vi "exponential fit.vi"() -> ()   [LabVIEW 2015]
uses:
  <vilib>/Utility/file.llb/Read Delimited Spreadsheet (DBL).vi
  <vilib>/Analysis/NI_AALPro.lvlib
  <vilib>/Analysis/NI_AALBase.lvlib
panel:
  out "Half Life (s)":dbl=-79.0458411255295
  out "Decay Plot":T1(graph)=[{"Best Exponential Fit"=[0.0, 1.0, 2.0, 3.0, 4.0, 5.0, 6.0, 7.0, 8.0, 9.0, 10.0, 11.0, 12.0, 13.0, 14.0, 15.0, 16.0, 17.0, 18.0, 19.0, 20.0, 21.0, 22.0, 23.0, 24.0, 25.0, 26.0, 27.0, 28.0, 29.0, 30.0, 31.0, 32.0, 33.0, 34.0, 35.0, 36.0, 37.0, 38.0, 39.0, 40.0, 41.0, 42.0, 43.0, 44.0, 45.0, 46.0, 47.0, 48.0, 49.0, 50.0, 51.0, 52.0, 53.0, 54.0, 55.0, 56.0, 57.0, 58.0, 59.0, 60.0, 61.0, 62.0, 63.0, 64.0, 65.0, 66.0, 67.0, 68.0, 69.0, 70.0, 71.0, 72.0, 73.0, 74.0, 75.0, 76.0, 77.0, 78.0, 79.0, 80.0, 81.0, 82.0, 83.0, 84.0, 85.0, 86.0, 87.0, 88.0, 89.0, 90.0, 91.0, 92.0, 93.0, 94.0, 95.0, 96.0, 97.0, 98.0, 99.0, 100.0, 101.0, 102.0, 103.0, 104.0, 105.0, 106.0, 107.0, 108.0, 109.0, 110.0, 111.0, 112.0, 113.0, 114.0, 115.0, 116.0, 117.0, 118.0, 119.0, 120.0, 121.0, 122.0, 123.0, 124.0, 125.0, 126.0, 127.0, 128.0, 129.0, 130.0, 131.0, 132.0, 133.0, 134.0, 135.0, 136.0, 137.0, 138.0, 139.0, 140.0, 141.0, 142.0, 143.0, 144.0, 145.0, 146.0, 147.0, 148.0, 149.0, 150.0, 151.0, 152.0, 153.0, 154.0, 155.0, 156.0, 157.0, 158.0, 159.0, 160.0, 161.0, 162.0, 163.0, 164.0, 165.0, 166.0, 167.0, 168.0, 169.0, 170.0, 171.0, 172.0, 173.0, 174.0, 175.0, 176.0, 177.0, 178.0, 179.0, 180.0, 181.0, 182.0, 183.0, 184.0, 185.0, 186.0, 187.0, 188.0, 189.0, 190.0, 191.0, 192.0, 193.0, 194.0, 195.0, 196.0, 197.0, 198.0, 199.0, 200.0, 201.0, 202.0, 203.0, 204.0, 205.0, 206.0, 207.0, 208.0, 209.0, 210.0, 211.0, 212.0, 213.0, 214.0, 215.0, 216.0, 217.0, 218.0, 219.0, 220.0, 221.0, 222.0, 223.0, 224.0, 225.0, 226.0, 227.0, 228.0, 229.0, 230.0, 231.0, 232.0, 233.0, 234.0, 235.0, 236.0, 237.0, 238.0, 239.0, 240.0, 241.0, 242.0, 243.0, 244.0, 245.0, 246.0, 247.0, 248.0, 249.0, 250.0, 251.0, 252.0, 253.0, 254.0, 255.0, 256.0, 257.0, 258.0, 259.0, 260.0, 261.0, 262.0, 263.0, 264.0, 265.0, 266.0, 267.0, 268.0, 269.0, 270.0, 271.0, 272.0, 273.0, 274.0, 275.0, 276.0, 277.0, 278.0, 279.0, 280.0, 281.0, 282.0, 283.0, 284.0, 285.0, 286.0, 287.0, 288.0, 289.0, 290.0, 291.0, 292.0, 293.0, 294.0, 295.0, 296.0, 297.0, 298.0, 299.0, 300.0], "all rows"=[0.0, 37.0, 51.0, 62.0, 64.0, 69.0, 55.0, 70.0, 52.0, 84.0, 66.0, 49.0, 62.0, 61.0, 55.0, 68.0, 51.0, 56.0, 55.0, 60.0, 46.0, 62.0, 45.0, 56.0, 63.0, 59.0, 49.0, 58.0, 53.0, 57.0, 63.0, 48.0, 55.0, 55.0, 49.0, 65.0, 45.0, 51.0, 39.0, 46.0, 45.0, 49.0, 47.0, 36.0, 56.0, 43.0, 55.0, 38.0, 37.0, 48.0, 48.0, 43.0, 57.0, 45.0, 37.0, 36.0, 47.0, 37.0, 28.0, 30.0, 42.0, 41.0, 39.0, 36.0, 42.0, 38.0, 39.0, 39.0, 32.0, 31.0, 33.0, 29.0, 37.0, 37.0, 27.0, 29.0, 24.0, 32.0, 31.0, 30.0, 37.0, 22.0, 41.0, 32.0, 32.0, 31.0, 33.0, 33.0, 30.0, 30.0, 30.0, 27.0, 19.0, 33.0, 27.0, 30.0, 27.0, 28.0, 29.0, 36.0, 35.0, 33.0, 22.0, 31.0, 12.0, 19.0, 14.0, 29.0, 28.0, 15.0, 17.0, 25.0, 18.0, 22.0, 26.0, 25.0, 17.0, 21.0, 20.0, 27.0, 21.0, 20.0, 20.0, 23.0, 31.0, 25.0, 24.0, 22.0, 14.0, 17.0, 13.0, 25.0, 16.0, 20.0, 28.0, 14.0, 23.0, 21.0, 23.0, 18.0, 26.0, 18.0, 22.0, 24.0, 10.0, 17.0, 13.0, 15.0, 12.0, 17.0, 19.0, 18.0, 13.0, 14.0, 22.0, 21.0, 12.0, 18.0, 18.0, 13.0, 9.0, 19.0, 21.0, 19.0, 12.0, 16.0, 11.0, 11.0, 14.0, 11.0, 20.0, 12.0, 7.0, 13.0, 9.0, 13.0, 15.0, 14.0, 19.0, 9.0, 13.0, 18.0, 12.0, 9.0, 10.0, 7.0, 9.0, 11.0, 9.0, 8.0, 7.0, 9.0, 13.0, 7.0, 23.0, 12.0, 15.0, 11.0, 10.0, 15.0, 6.0, 13.0, 10.0, 8.0, 4.0, 13.0, 15.0, 8.0, 12.0, 8.0, 12.0, 4.0, 10.0, 16.0, 13.0, 12.0, 12.0, 8.0, 6.0, 14.0, 10.0, 7.0, 13.0, 9.0, 10.0, 13.0, 7.0, 12.0, 8.0, 6.0, 3.0, 9.0, 6.0, 8.0, 12.0, 10.0, 7.0, 9.0, 8.0, 11.0, 9.0, 4.0, 1.0, 3.0, 11.0, 4.0, 5.0, 3.0, 8.0, 8.0, 13.0, 4.0, 8.0, 5.0, 6.0, 5.0, 5.0, 4.0, 6.0, 9.0, 6.0, 5.0, 5.0, 4.0, 5.0, 6.0, 3.0, 8.0, 9.0, 6.0, 8.0, 7.0, 4.0, 4.0, 7.0, 9.0, 4.0, 7.0, 4.0, 5.0, 3.0, 8.0, 6.0, 7.0, 5.0, 3.0, 5.0, 6.0, 4.0, 6.0, 6.0, 3.0, 1.0, 5.0, 8.0, 7.0, 3.0, 2.0, 3.0, 6.0, 5.0]}, {"Best Exponential Fit"=[0.0, 1.0, 2.0, 3.0, 4.0, 5.0, 6.0, 7.0, 8.0, 9.0, 10.0, 11.0, 12.0, 13.0, 14.0, 15.0, 16.0, 17.0, 18.0, 19.0, 20.0, 21.0, 22.0, 23.0, 24.0, 25.0, 26.0, 27.0, 28.0, 29.0, 30.0, 31.0, 32.0, 33.0, 34.0, 35.0, 36.0, 37.0, 38.0, 39.0, 40.0, 41.0, 42.0, 43.0, 44.0, 45.0, 46.0, 47.0, 48.0, 49.0, 50.0, 51.0, 52.0, 53.0, 54.0, 55.0, 56.0, 57.0, 58.0, 59.0, 60.0, 61.0, 62.0, 63.0, 64.0, 65.0, 66.0, 67.0, 68.0, 69.0, 70.0, 71.0, 72.0, 73.0, 74.0, 75.0, 76.0, 77.0, 78.0, 79.0, 80.0, 81.0, 82.0, 83.0, 84.0, 85.0, 86.0, 87.0, 88.0, 89.0, 90.0, 91.0, 92.0, 93.0, 94.0, 95.0, 96.0, 97.0, 98.0, 99.0, 100.0, 101.0, 102.0, 103.0, 104.0, 105.0, 106.0, 107.0, 108.0, 109.0, 110.0, 111.0, 112.0, 113.0, 114.0, 115.0, 116.0, 117.0, 118.0, 119.0, 120.0, 121.0, 122.0, 123.0, 124.0, 125.0, 126.0, 127.0, 128.0, 129.0, 130.0, 131.0, 132.0, 133.0, 134.0, 135.0, 136.0, 137.0, 138.0, 139.0, 140.0, 141.0, 142.0, 143.0, 144.0, 145.0, 146.0, 147.0, 148.0, 149.0, 150.0, 151.0, 152.0, 153.0, 154.0, 155.0, 156.0, 157.0, 158.0, 159.0, 160.0, 161.0, 162.0, 163.0, 164.0, 165.0, 166.0, 167.0, 168.0, 169.0, 170.0, 171.0, 172.0, 173.0, 174.0, 175.0, 176.0, 177.0, 178.0, 179.0, 180.0, 181.0, 182.0, 183.0, 184.0, 185.0, 186.0, 187.0, 188.0, 189.0, 190.0, 191.0, 192.0, 193.0, 194.0, 195.0, 196.0, 197.0, 198.0, 199.0, 200.0, 201.0, 202.0, 203.0, 204.0, 205.0, 206.0, 207.0, 208.0, 209.0, 210.0, 211.0, 212.0, 213.0, 214.0, 215.0, 216.0, 217.0, 218.0, 219.0, 220.0, 221.0, 222.0, 223.0, 224.0, 225.0, 226.0, 227.0, 228.0, 229.0, 230.0, 231.0, 232.0, 233.0, 234.0, 235.0, 236.0, 237.0, 238.0, 239.0, 240.0, 241.0, 242.0, 243.0, 244.0, 245.0, 246.0, 247.0, 248.0, 249.0, 250.0, 251.0, 252.0, 253.0, 254.0, 255.0, 256.0, 257.0, 258.0, 259.0, 260.0, 261.0, 262.0, 263.0, 264.0, 265.0, 266.0, 267.0, 268.0, 269.0, 270.0, 271.0, 272.0, 273.0, 274.0, 275.0, 276.0, 277.0, 278.0, 279.0, 280.0, 281.0, 282.0, 283.0, 284.0, 285.0, 286.0, 287.0, 288.0, 289.0, 290.0, 291.0, 292.0, 293.0, 294.0, 295.0, 296.0, 297.0, 298.0, 299.0, 300.0], "all rows"=[64.13781261084702, 63.5778515552424, 63.02277929099237, 62.4725531360556, 61.92713078103027, 61.386470285900664, 60.85053007681219, 60.31926894287464, 59.79264603299326, 59.27062085272752, 58.75315326117729, 58.2402034678963, 57.73173202983239, 57.22769984829459, 56.72806816594664, 56.23279856382675, 55.7418529583934, 55.255193598596954, 54.772783062976735, 54.29458425678358, 53.82056040912744, 53.35067507014988, 52.88489210822131, 52.42317570716263, 51.9654903634912, 51.51180088369078, 51.062072381505345, 50.616270275256525, 50.17436028518449, 49.73630843081198, 49.30208102833139, 48.87164468801474, 48.444966311646056, 48.02201308997645, 47.602752500201134, 47.18715230345869, 46.77518054235202, 46.36680553849099, 45.961995890056606, 45.5607204693863, 45.16294842058041, 44.768649157129566, 44.37779235956271, 43.990347973115696, 43.606286205420254, 43.22557752421314, 42.84819265506523, 42.47410257913049, 42.103278530914565, 41.735691996062904, 41.371314709168146, 41.01011865159666, 40.65207604933406, 40.29715937084954, 39.945341324978855, 39.59659485882577, 39.25089315568183, 38.90820963296433, 38.56851794017224, 38.231791956859986, 37.89800579062894, 37.56713377513646, 37.23915046812222, 36.9140306494519, 36.59174931917791, 36.27228169561693, 35.955603213444455, 35.641689521805766, 35.33051648244354, 35.022060167841694, 34.716296859385544, 34.41320304553794, 34.11275542003135, 33.814930880075764, 33.5197065245822, 33.22705965240172, 32.93696776057986, 32.64940854262626, 32.36435988679942, 32.081799874406435, 31.80170677811755, 31.52405906029545, 31.248835371339144, 30.976014548042297, 30.705575611965884, 30.437497767825064, 30.171760401890133, 29.908343080401455, 29.6472255479982, 29.38838772616083, 29.131809711667145, 28.87747177506188, 28.62535435913957, 28.375438077440727, 28.127703712761132, 27.88213221567412, 27.638704703065812, 27.397402456683064, 27.158206921694173, 26.921099705262083, 26.686062575130116, 26.453077458219944, 26.22212643924194, 25.99319175931753, 25.76625581461369, 25.54130115498924, 25.318310482653082, 25.09726665083406, 24.878152662462483, 24.660951668863124, 24.445646968459673, 24.232222005490456, 24.020660368735403, 23.81094579025409, 23.603062144134853, 23.396993445254783, 23.192723848050534, 22.990237645299924, 22.789519266914095, 22.5905532787403, 22.393324381375056, 22.19781740898775, 22.004017328154415, 21.81190923670179, 21.621478362561408, 21.43271006263369, 21.245589821661973, 21.060103251116406, 20.876236088087477, 20.693974194189344, 20.513303554472618, 20.33421027634673, 20.156680588511637, 19.980700839898894, 19.80625749862196, 19.633337150935677, 19.461926500204818, 19.292012365881643, 19.1235816824924, 18.95662149863264, 18.791118975971358, 18.627061388263773, 18.46443612037273, 18.303230667298713, 18.14343263321824, 17.98502973053069, 17.82800977891349, 17.67236070438547, 17.51807053837847, 17.365127416817018, 17.21351957920602, 17.06323536772649, 16.914263226339084, 16.766591699895518, 16.620209433257738, 16.475105170424754, 16.331267753667138, 16.18868612266904, 16.047349313677696, 15.907246458660419, 15.768366784468851, 15.63069961201061, 15.494234355428098, 15.358960521284528, 15.22486770775703, 15.091945603836784, 14.960183988536187, 14.829572730102917, 14.70010178524083, 14.571761198337706, 14.444541100699707, 14.318431709792536, 14.19342332848921, 14.069506344324399, 13.946671228755278, 13.824908536428856, 13.704208904455646, 13.584563051689733, 13.465961778015094, 13.348395963638168, 13.231856568386588, 13.116334631014038, 13.001821268511183, 12.888307675422622, 12.775785123169783, 12.664244959379758, 12.553678607219965, 12.444077564738649, 12.33543340421113, 12.227737771491745, 12.120982385371464, 12.015159036941126, 11.910259588960184, 11.80627597523103, 11.703200199978731, 11.601024337236193, 11.499740530234723, 11.399340990799846, 11.29981799875247, 11.201163901315239, 11.103371112524059, 11.0064321126448, 10.910339447595062, 10.815085728370983, 10.720663630479093, 10.627065893373075, 10.534285319895478, 10.442314775724295, 10.351147188824374, 10.260775548903611, 10.171192906873902, 10.08239237431679, 9.994367122953799, 9.907110384121347, 9.820615448250305, 9.734875664350048, 9.64988443949703, 9.565635238327836, 9.482121582536637, 9.399337050377044, 9.31727527616832, 9.235929949805886, 9.155294816276106, 9.075363675175318, 8.996130380233053, 8.917588838839418, 8.83973301157661, 8.762556911754515, 8.686054604950373, 8.610220208552438, 8.535047891307654, 8.460531872873242, 8.386666423372251, 8.313445862952936, 8.24086456135202, 8.168916937461757, 8.097597458900772, 8.026900641588663, 7.956821049324283, 7.887353293367743, 7.818492032026039, 7.750231970242311, 7.682567859188677, 7.615494495862627, 7.549006722686946, 7.483099427113111, 7.417767541228186, 7.353006041365104, 7.288809947716384, 7.225174323951217, 7.1620942768358775, 7.099564955857467, 7.0375815528509325, 6.976139301629357, 6.915233477617446, 6.8548593974882435, 6.795012418803012, 6.735687939654249, 6.676881398311831, 6.618588272872233, 6.560804080910827, 6.5035243791372, 6.446744763053503, 6.39046086661575, 6.334668361898104, 6.2793629587600845, 6.224540404516675, 6.1701964836113135, 6.116327017291741, 6.062927863288686, 6.00999491549733, 5.957524103661581, 5.9055113930610945, 5.8539527842010175, 5.802844312504456, 5.7521820480076205, 5.701962095057627, 5.652180592012944, 5.6028337109464665, 5.553917657351147, 5.505428669848236, 5.457363019898041, 5.409717011513234, 5.3624869809746345, 5.315669296549506, 5.2692603582122866, 5.223256597367765, 5.177654476576681, 5.132450489283706, 5.087641159547824, 5.043223041775032, 4.999192720453404, 4.955546809890459, 4.912281953952806, 4.869394825808094, 4.8268821276691805, 4.784740590540557, 4.742966973966982, 4.701558065784304, 4.6605106818724655, 4.619821665910661]}]
  in  "Path 2":path=path "C:/Users/senkoa/Desktop/PHYS434/week8/constant data"
  in  "Path":path=path "C:/Users/senkoa/Desktop/PHYS434/week8/data"
  out "Constant Rate":T2(graph)={"X Values"=[2.0714285714285716, 6.214285714285714, 10.357142857142858, 14.5, 18.642857142857142, 22.785714285714285, 26.928571428571427, 31.071428571428573, 35.214285714285715, 39.357142857142854, 43.5, 47.642857142857146, 51.785714285714285, 55.92857142857143], "Histogram: h(x)"=[1, 0, 0, 0, 0, 1, 2, 21, 13, 30, 27, 14, 10, 2]}
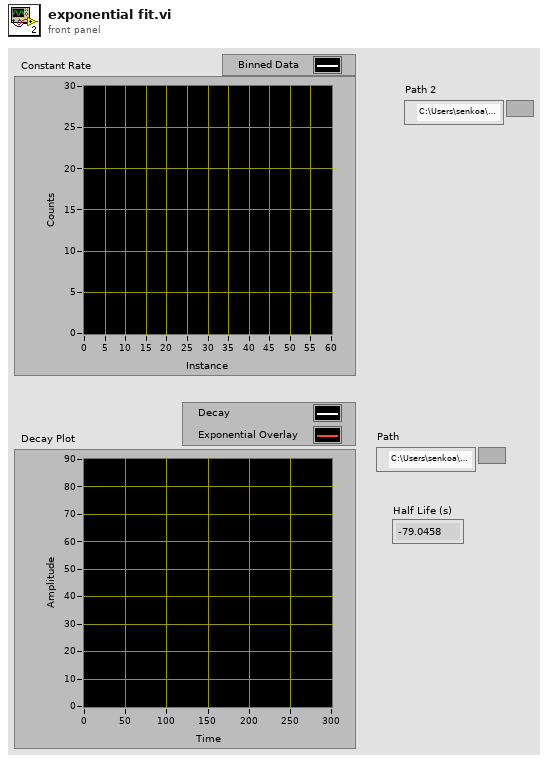
[diagram p1: front panel]
types:
  T1 = cluster{"Best Exponential Fit":dbl[], "all rows":dbl[]}[]
  T2 = cluster{"X Values":dbl[], "Histogram: h(x)":i32[]}
  T3 = cluster{"all rows":dbl[], "Best Exponential Fit":dbl[]}
  T4 = cluster{"all rows":dbl[], "Best Exponential Fit":dbl[]}[]
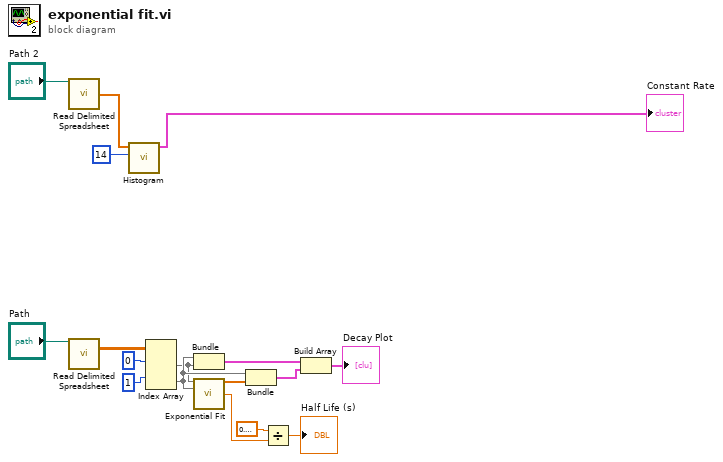
[diagram p0: block diagram]
diagram:
  n1 = call-poly <vilib>:"Read Delimited Spreadsheet.vi"("file path (dialog if empty)"="Path 2") -> ("first row"=w2:dbl[])  [unwired: 9 in, 5 out]
  n2 = call-poly <vilib>:"Read Delimited Spreadsheet.vi"("file path (dialog if empty)"="Path") -> ("all rows"=w15:dbl[][])  [unwired: 9 in, 5 out]
  n3 = call <vilib>:"Histogram.vi"("intervals"=14, "X"=w2) -> ("Histogram Graph"=→"Constant Rate":T2)  [unwired: 6 in, 3 out]
  n4 = Index Array(array=w15, index (row) #1=0 ("index (row)"), index (row) #2=1 ("index (row)")) -> (element #1=w7:dbl[], element #2=w8:dbl[])  [unwired: 2 in]
  n5 = Bundle("all rows"=w8, "all rows"=w7) -> (w12:cluster{"all rows":dbl[], "all rows":dbl[]})  [unwired: 1 in]
  n6 = call <vilib>:"Exponential Fit.vi"("Y"=w7, "X"=w8) -> ("Best Exponential Fit"=w9:dbl[], "damping"=w6:dbl)  [unwired: 8 in, 4 out]
  n7 = Bundle("all rows"=w8, "Best Exponential Fit"=w9) -> (w11:T3)  [unwired: 1 in]
  n8 = Divide(x=0.6931471805599453, y=w6) -> (x/y=→"Half Life (s)":dbl)
  n9 = Build Array(w12, w11) -> (→"Decay Plot":T4)
